vi "Server and Client.vi"   [LabVIEW 2015, in "AguaClara Library.lvlib"]
uses:
  AguaClara Library.lvlib
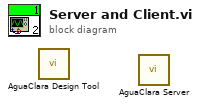
[diagram p0: block diagram]
diagram:
  n1 = call "AguaClara Design Tool.vi"() -> ()  [unwired: 12 in]
  n2 = call "AguaClara Server.vi"() -> ()  [unwired: 12 in]
